vi "PAM CC Read Write TCP.vi"(3 "Error In":errorcluster {"code" format="%.0x"}, 4 "ID In":refnum<k5>, 5 "Command":string) -> (0 "Error Out":errorcluster, 1 "ID Out":refnum<k5>, 2 "Response":string)   [LabVIEW 2020]
doc: "Launches the Instrument I/O Assistant, which you can use to communicate with message-based instruments and graphically parse the response. For example you can communicate with an instrument that uses a serial, Ethernet, or GPIB interface."
uses:
  CRC-16R Table.ctl
  PAM Library.lvlib
panel:
  out "Response":string
  out "Read Loop Iteration":i32
  out "Command and CRC":string
  out "CRC":string
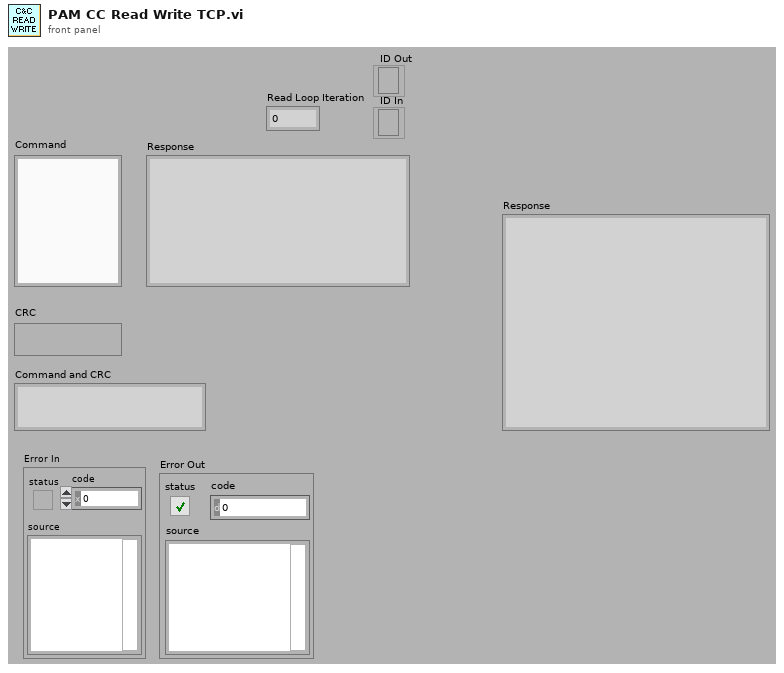
[diagram p1: front panel]
types:
  T1 = typedef "PAM Library.lvlib/CRC-16R Table.ctl" = u16[]
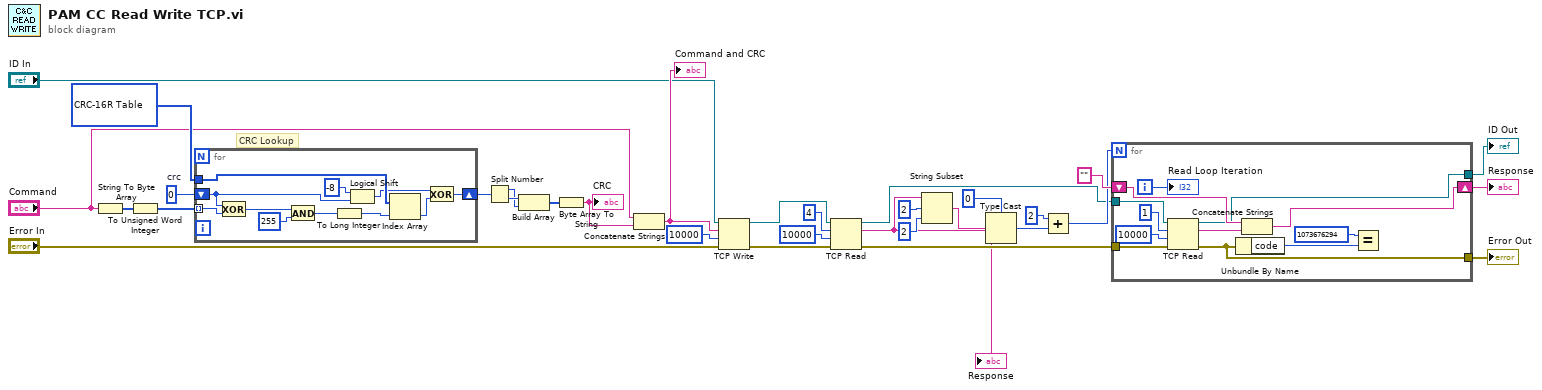
[diagram p0: block diagram]
diagram:
  w29 = u16 0  # crc
  # "CRC Lookup"
  n1 = String To Byte Array(string="Command") -> (unsigned byte array=w28:u8[])
  n2 = To Unsigned Word Integer(number=w28) -> (unsigned 16bit integer=w27:u16[])
  n3 = for {
    shift-right: [w39] -> w31
    shift-left: w29 -> [w38]
    tunnel: T1 [0, 49345, 49537, 320, 49921, 960, 640, 49729, 50689, 1728, 1920, 51009, 1280, 50625, 50305, 1088, 52225, 3264, 3456, 52545, 3840, 53185, 52865, 3648, 2560, 51905, 52097, 2880, 51457, 2496, 2176, 51265, 55297, 6336, 6528, 55617, 6912, 56257, 55937, 6720, 7680, 57025, 57217, 8000, 56577, 7616, 7296, 56385, 5120, 54465, 54657, 5440, 55041, 6080, 5760, 54849, 53761, 4800, 4992, 54081, 4352, 53697, 53377, 4160, 61441, 12480, 12672, 61761, 13056, 62401, 62081, 12864, 13824, 63169, 63361, 14144, 62721, 13760, 13440, 62529, 15360, 64705, 64897, 15680, 65281, 16320, 16000, 65089, 64001, 15040, 15232, 64321, 14592, 63937, 63617, 14400, 10240, 59585, 59777, 10560, 60161, 11200, 10880, 59969, 60929, 11968, 12160, 61249, 11520, 60865, 60545, 11328, 58369, 9408, 9600, 58689, 9984, 59329, 59009, 9792, 8704, 58049, 58241, 9024, 57601, 8640, 8320, 57409, 40961, 24768, 24960, 41281, 25344, 41921, 41601, 25152, 26112, 42689, 42881, 26432, 42241, 26048, 25728, 42049, 27648, 44225, 44417, 27968, 44801, 28608, 28288, 44609, 43521, 27328, 27520, 43841, 26880, 43457, 43137, 26688, 30720, 47297, 47489, 31040, 47873, 31680, 31360, 47681, 48641, 32448, 32640, 48961, 32000, 48577, 48257, 31808, 46081, 29888, 30080, 46401, 30464, 47041, 46721, 30272, 29184, 45761, 45953, 29504, 45313, 29120, 28800, 45121, 20480, 37057, 37249, 20800, 37633, 21440, 21120, 37441, 38401, 22208, 22400, 38721, 21760, 38337, 38017, 21568, 39937, 23744, 23936, 40257, 24320, 40897, 40577, 24128, 23040, 39617, 39809, 23360, 39169, 22976, 22656, 38977, 34817, 18624, 18816, 35137, 19200, 35777, 35457, 19008, 19968, 36545, 36737, 20288, 36097, 19904, 19584, 35905, 17408, 33985, 34177, 17728, 34561, 18368, 18048, 34369, 33281, 17088, 17280, 33601, 16640, 33217, 32897, 16448] ("CRC-16R table") -> [w42]
    tunnel: w27 -> [w36] mode=indexing
    n4 = Exclusive Or(1:w36, 2:w38) -> (0:w35:u16)
    n5 = And(x=w35, y=u16 255) -> (x .and. y?=w41:u16)
    n6 = To Long Integer(number=w41) -> (32bit integer=w33:i32)
    n7 = Logical Shift(y=-8, x=w38) -> (x << y=w37:u16)
    n8 = Index Array(array=w42, index=w33) -> (element=w40:u16)
    n9 = Exclusive Or(1:w40, 2:w37) -> (0:w39:u16)
  }
  n10 = Split Number(x=w31) -> (hi(x)=w23:u8, lo(x)=w24:u8)
  n11 = Build Array(w24, w23) -> (w26:u8[])
  n12 = Byte Array To String(unsigned byte array=w26) -> (string=w13:string)
  "CRC" <- w13
  n13 = Concatenate Strings("Command", w13) -> (w11:string)
  "Command and CRC" <- w11
  n14 = TCP Write(connection ID="ID In", data in=w11, error in (no error)="Error In", 9:10000 ("timeout ms (25000)")) -> (connection ID out=w4:refnum<k5>, error out=w8:errorcluster)  [unwired: 1 out]
  n15 = TCP Read(connection ID=w4, bytes to read=4 ("byte count (0)"), error in (no error)=w8, 9:10000 ("timeout ms (25000)")) -> (connection ID out=w3:refnum<k5>, data out=w5:string, error out=w7:errorcluster)  [unwired: 1 in]
  "Response" <- w5
  n16 = String Subset(string=w5, offset (0)=2, length (rest)=2 ("length (rest)")) -> (substring=w17:string)
  n17 = Type Cast(type=u8 0, x=w17) -> (*(type *) &x=w16:u8)
  n18 = Add(x=u8 2, y=w16) -> (x+y=w14:u8)
  n19 = for {
    N: w14 -> [_]
    shift-left: "" -> [w53]
    shift-right: [w52] -> w25
    tunnel: w7 -> [w49]
    tunnel: [w46] -> w21
    tunnel: [w47] -> w12
    tunnel: w3 -> [w45]
    i -> [w51]
    n20 = TCP Read(connection ID=w45, bytes to read=1 ("byte count (0)"), error in (no error)=w49, 9:10000 ("timeout ms (25000)")) -> (connection ID out=w47:refnum<k5>, data out=w48:string, error out=w46:errorcluster)  [unwired: 1 in]
    n21 = Unbundle By Name(w46) -> ("code"=w55:i32)
    n22 = Concatenate Strings(w53, w48) -> (w52:string)
    n23 = Equal?(x=1073676294, y=w55) -> ()  [unwired: 1 out]
    "Read Loop Iteration" <- w51
  }
  "Response" <- w25
  "Error Out" <- w21
  "ID Out" <- w12
